vi "Word Report.vi"(6 "מק\"ט המכלל":string, 7 "עבר/נכשל":string="עבר/נכשל", 8 "מספר סידורי":string, 9 "שם הצב\"ד":string="שם הצב\"ד", 10 "מפעיל":string="ANS", 11 "Array":string[][](array[string])=[["Content", "Results", "Range", "Pass/Fail", "11"], ["Content", "Results", "Range", "Pass/Fail", "22"], ["Content", "Results", "Range", "Pass/Fail", "33"], ["Content", "Results", "Range", "Pass/Fail", "44"], ["Content", "Results", "Range", "Pass/Fail", "55"], ["55", "Content", "Results", "Range", "Pass/Fail"]]) -> ()   [LabVIEW 2015]
uses:
  <vilib>/addons/_office/_exclsub.llb/font.ctl
  <vilib>/addons/_office/word.llb/Word Easy Table (str).vi
  <vilib>/addons/_office/word.llb/Word Edit Cell ([str]).vi
  <vilib>/addons/_office/NI_ReportGenerationToolkit.lvlib
  <vilib>/Utility/NIReport.llb/Word/NI_Word.lvclass
panel:
  in  "start (0, 0)":cluster{"row":i32, "column":i32}={"row"=1, "column"=4}
  in  "value 3":string[][](array[string])
  in  "new element/subarray 3":string[](array[string])
  in  "new element/subarray":string[](array[string])
  in  "value":string[][](array[string])
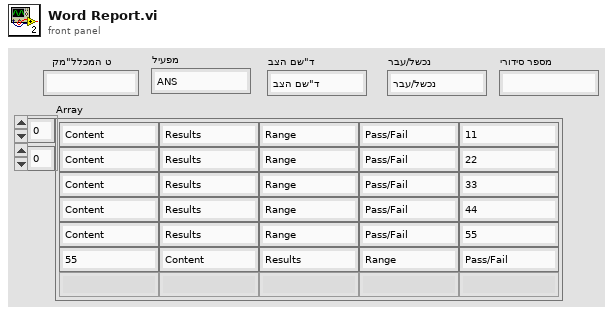
[diagram p1: front panel]
types:
  T1 = typedef "NI_ReportGenerationToolkit.lvlib/font.ctl" = cluster{"font name":string, "font size":dbl, "bold":u16, "italic":u16, "underline":u16, "strike through":u16, "font color":u32}
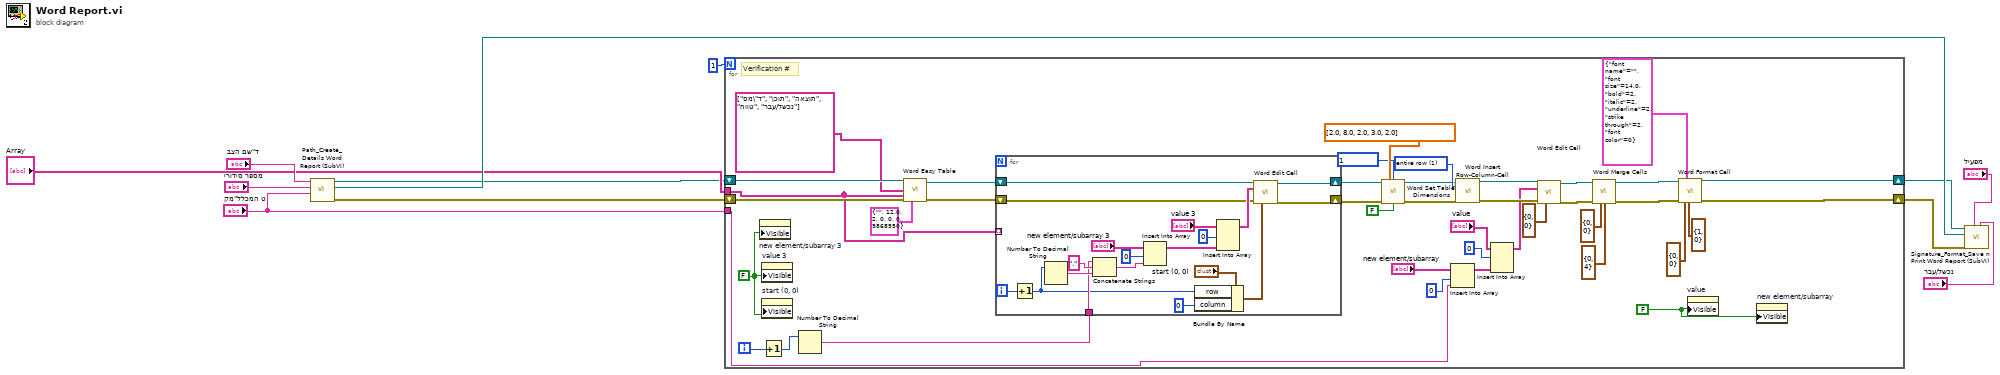
[diagram p0: block diagram]
diagram:
  n1 = call "Path_Create_Details Word Report (SubVI).vi"("שם ומק\"ט המכלל"="מק\"ט המכלל", "מספר סידורי"="מספר סידורי", "שם הצב\"ד"="שם הצב\"ד") -> ("error out"=w4:errorcluster, "Path"=w11:path, "NI_report out"=w5:refnum<class "NI_report.lvclass">)  [unwired: 6 in]
  n2 = for {
    N: 1 -> [_]
    shift-right: [w21] -> w9
    shift-left: w4 -> [w53]
    shift-right: [w22] -> w10
    shift-left: w5 -> [w52]
    tunnel: "Array" -> [w25]
    tunnel: "מק\"ט המכלל" -> [w13]
    i -> [w32]
    w33 = FALSE
    w39 = FALSE
    w51 = u16 1 items=["shift cells right", "entire row", "entire column"] ("mode (entire column)")
    # "Verification #"
    n3 = property on="new element/subarray 3" class="Arr (strict)"("Visible"=w33) -> ()  [unwired: 2 in, 2 out]
    n4 = property on="value 3" class="Arr (strict)"("Visible"=w33) -> ()  [unwired: 2 in, 2 out]
    n5 = property on="start (0, 0)" class="Clust (strict)"("Visible"=w33) -> ()  [unwired: 2 in, 2 out]
    n6 = Increment(x=w32) -> (x+1=w31:i32)
    n7 = Number To Decimal String(number=w31) -> (decimal integer string=w29:string)  [unwired: 1 in]
    n8 = call-poly <vilib>:"Word Easy Table.vi"("report in"=w52, "column headers"=string[] ["מס\"ד", "תוכן", "תוצאה", "טווח", "עבר/נכשל"], "data"=w25, "error in (no error)"=w53, "font"=T1 {"font name"="", "font size"=12.0, "bold"=2, "italic"=0, "underline"=0, "strike through"=0, "font color"=9868950}) -> ("report out"=w35:refnum<class "NI_report.lvclass">, "error out"=w34:errorcluster)  [unwired: 8 in, 1 out]
    n9 = for {
      shift-right: [w59] -> w20
      shift-left: w35 -> [w54]
      shift-right: [w58] -> w19
      shift-left: w34 -> [w55]
      tunnel: w29 -> [w63]
      tunnel: w25 -> [_] mode=indexing
      i -> [w60]
      n10 = Increment(x=w60) -> (x+1=w61:i32)
      n11 = Number To Decimal String(number=w61) -> (decimal integer string=w64:string)  [unwired: 1 in]
      n12 = Concatenate Strings(w63, ".", w64) -> (w66:string)
      n13 = Insert Into Array(array="new element/subarray 3", index=0, new element=w66) -> (w71:string[])
      n14 = Bundle By Name(cluster="start (0, 0)", "row"=w61, "column"=0) -> (w56:cluster{"row":i32, "column":i32})
      n15 = Insert Into Array(array="value 3", index (row)=0 ("disabled index (col)"), new element=w71) -> (w57:string[][])  [unwired: 1 in]
      n16 = call-poly <vilib>:"Word Edit Cell.vi"("report in"=w54, "value"=w57, "error in (no error)"=w55, "start (0, 0)"=w56) -> ("report out"=w59:refnum<class "NI_report.lvclass">, "error out"=w58:errorcluster)  [unwired: 10 in]
    }
    n17 = call <vilib>:"Word Set Table Dimensions.vi"("report in"=w20, "table column widths"=sgl[] [2.0, 8.0, 2.0, 3.0, 2.0], "measurement system"=u16 1, "error in (no error)"=w19, "fit to page width? (F)"=FALSE) -> ("report out"=w17:refnum<class "NI_report.lvclass">, "error out"=w18:errorcluster)  [unwired: 9 in]
    n18 = Insert Into Array(array="new element/subarray", index=0, new element=w13) -> (w43:string[])
    n19 = call <vilib>:"Word Insert Row-Column-Cell.vi"("report in"=w17, "mode (entire column)"=w51, "error in (no error)"=w18) -> ("report out"=w50:refnum<class "NI_report.lvclass">, "error out"=w49:errorcluster)  [unwired: 11 in]
    n20 = Insert Into Array(array="value", index (row)=0, new element=w43) -> (w41:string[][])  [unwired: 1 in]
    n21 = call-poly <vilib>:"Word Edit Cell.vi"("report in"=w50, "value"=w41, "error in (no error)"=w49, "start (0, 0)"=cluster{"row":i32, "column":i32} {"row"=0, "column"=0}) -> ("report out"=w27:refnum<class "NI_report.lvclass">, "error out"=w26:errorcluster)  [unwired: 10 in]
    n22 = call <vilib>:"Word Merge Cells.vi"("report in"=w27, "error in (no error)"=w26, "start (0, 0)"=cluster{"start row":i32, "start column":i32} {"start row"=0, "start column"=0}, "end"=cluster{"end row":i32, "end column":i32} {"end row"=0, "end column"=4}) -> ("report out"=w24:refnum<class "NI_report.lvclass">, "error out"=w23:errorcluster)  [unwired: 10 in]
    n23 = call <vilib>:"Word Format Cell.vi"("report in"=w24, "font"=T1 {"font name"="", "font size"=14.0, "bold"=2, "italic"=2, "underline"=2, "strike through"=2, "font color"=0}, "error in (no error)"=w23, "start (-1, -1)"=cluster{"start row":i32, "start column":i32} {"start row"=1, "start column"=0}, "end (-1, -1)"=cluster{"end row":i32, "end column":i32} {"end row"=0, "end column"=0}) -> ("report out"=w22:refnum<class "NI_report.lvclass">, "error out"=w21:errorcluster)  [unwired: 9 in]
    n24 = property on="value" class="Arr (strict)"("Visible"=w39) -> ()  [unwired: 2 in, 2 out]
    n25 = property on="new element/subarray" class="Arr (strict)"("Visible"=w39) -> ()  [unwired: 2 in, 2 out]
  }
  n26 = call "Signature_Format_Save n Print Word Report (SubVI).vi"("עבר/נכשל"="עבר/נכשל", "מפעיל"="מפעיל", "error in (no error)"=w9, "Path"=w11, "NI_report in"=w10) -> ()  [unwired: 7 in]
